vi "sample palette.vi"() -> ()   [LabVIEW 2013]
uses:
  Controls/Add.ctl
  Controls/Remove.ctl
  Controls/Configure.ctl
  Controls/Move One Left.ctl
  Controls/Move One Right.ctl
  Controls/Move All Left.ctl
  Controls/Move All Right.ctl
  Controls/DCAF UI Elements.lvlib
panel:
  in  "Move All Right":T1
  in  "Add 2":T2
  in  "Move One Right":T3
  in  "Move One Left":T4
  in  "Configure":T5
  in  "Remove":T6
  in  "Add":T7
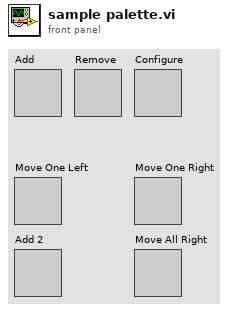
[diagram p1: front panel]
types:
  T1 = typedef "DCAF UI Elements.lvlib/Move All Right.ctl" = bool
  T2 = typedef "DCAF UI Elements.lvlib/Move All Left.ctl" = bool
  T3 = typedef "DCAF UI Elements.lvlib/Move One Right.ctl" = bool
  T4 = typedef "DCAF UI Elements.lvlib/Move One Left.ctl" = bool
  T5 = typedef "DCAF UI Elements.lvlib/Configure.ctl" = bool
  T6 = typedef "DCAF UI Elements.lvlib/Remove.ctl" = bool
  T7 = typedef "DCAF UI Elements.lvlib/Add.ctl" = bool
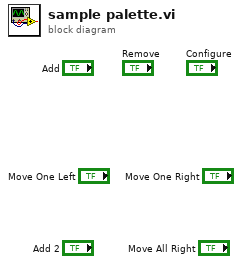
[diagram p0: block diagram]
diagram:
